vi "move_and_rename.vi"(6 "overwrite (F)":bool, 7 "file_to_move":path, 8 "error in (no error)":errorcluster, 9 "mark":string, 11 "target path":path) -> (0 "error out":errorcluster, 5 "renamed_file":path)   [LabVIEW 2015]
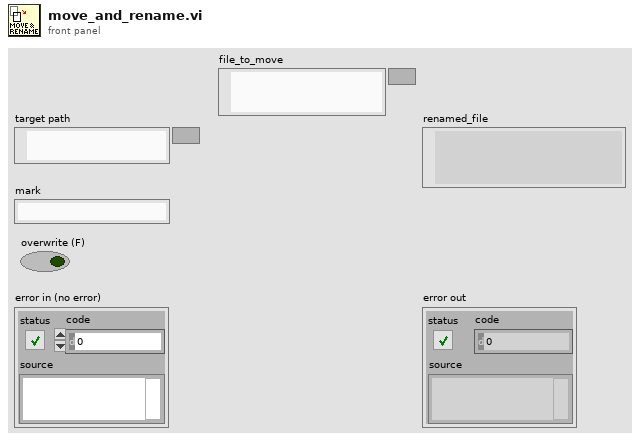
[diagram p1: front panel]
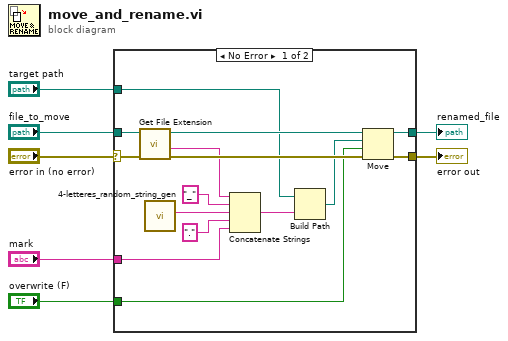
[diagram p0: block diagram]
diagram:
  n1 = case shown="No Error" "error in (no error)" {
    selector: "error in (no error)" -> [w19 w23]
    tunnel: "file_to_move" -> [w22 w24]
    tunnel: [w14 w23] -> w3
    tunnel: [w13 w24] -> w6
    tunnel: "mark" -> [w18 _]
    tunnel: "overwrite (F)" -> [w9 _]
    tunnel: "target path" -> [w8 _]
    frame No Error {
      n2 = call <vilib>:"Get File Extension.vi"("error in (no error)"=w19, "file"=w22) -> ("error out"=w21:errorcluster, "filename without extension"=w12:string, "dup file"=w15:path)  [unwired: 5 in, 2 out]
      n3 = call "4-letteres_random_string_gen.vi"() -> ("4-letters random string"=w10:string)  [unwired: 11 in]
      n4 = Concatenate Strings(w12, "_" ("string"), w10, ".", w18) -> (w16:string)
      n5 = Build Path(base path=w8, name or relative path=w16) -> (appended path=w17:path)
      n6 = Move(source path=w15, error in=w21, 9:w9, 10:w17) -> (error out=w14:errorcluster, 3:w13:path)  [unwired: 1 in, 1 out]
    }
    frame Error {
    }
  }
  "error out" <- w3
  "renamed_file" <- w6
